vi "main.vi"() -> ()   [LabVIEW 2015]
uses:
  <vilib>/Utility/NIReport.llb/NI_report.lvclass
  Agilent 3352X Series/Agilent 3352X Series.lvlib
panel:
  out "消息":string
  in  "幅值线性度":bool=TRUE
  in  "幅频响应":bool=TRUE
  in  "参考灵敏度":bool=TRUE
  out "已连接":bool
  in  "连接设备":bool
  in  "原始记录模板":string(combo)="外接电源型加速度计(公开).xls"
  in  "被测通道":tag="PXI2Slot3/ai1:3" caption="标准通道"
  in  "方向选择":string(combo)="Z向"
  in  "参考通道":tag="PXI2Slot3/ai0" caption="标准通道"
  in  "信号发生器(33XXX系列)":refnum<visa-resource-name>="USB0::0x0957::0x2C07::MY52810975::INSTR"
  in  "保存":bool
  in  "停止":bool
  in  "测量":bool
  # "加速度传感器校准软件"
  # "仪器设置"
  # "连接"
  # "参数配置"
  # "控制"
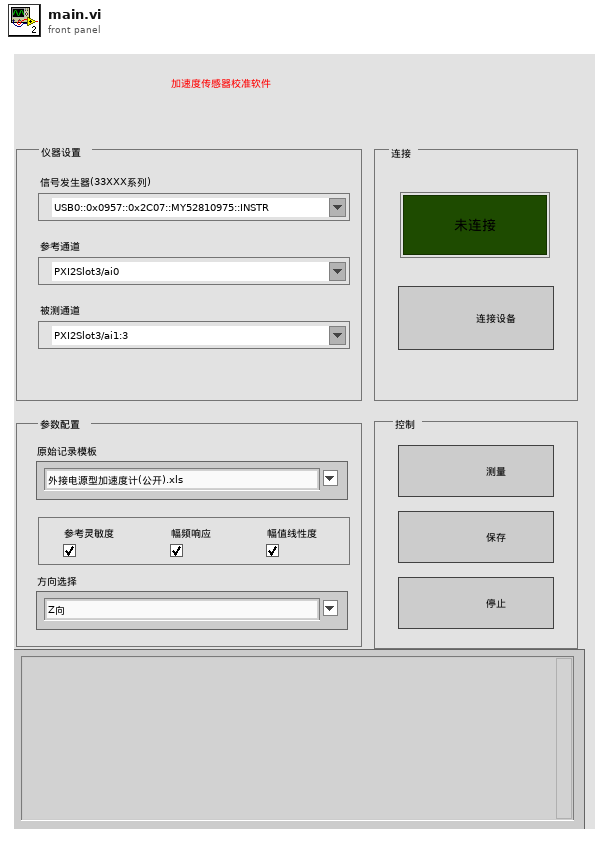
[diagram p1: front panel]
types:
  T1 = typedef "测试状态.ctl" = enum16{"idle", "路径配置", "参考灵敏度", "幅频响应", "幅值线性度", "结束", "停止"}
  T2 = typedef "句柄.ctl" = cluster{"33XXX":refnum<visa-resource-name>, "参考通道":tag, "被测通道":tag, "模板":refnum<class "NI_report.lvclass">}
  T3 = enum16{"Standard Report", "HTML", "Word", "Excel"}
  T4 = enum16{"maximized", "minimized", "normal", "no change"}
  T5 = enum8{"Enabled", "Disabled", "Disabled and Grayed Out"}
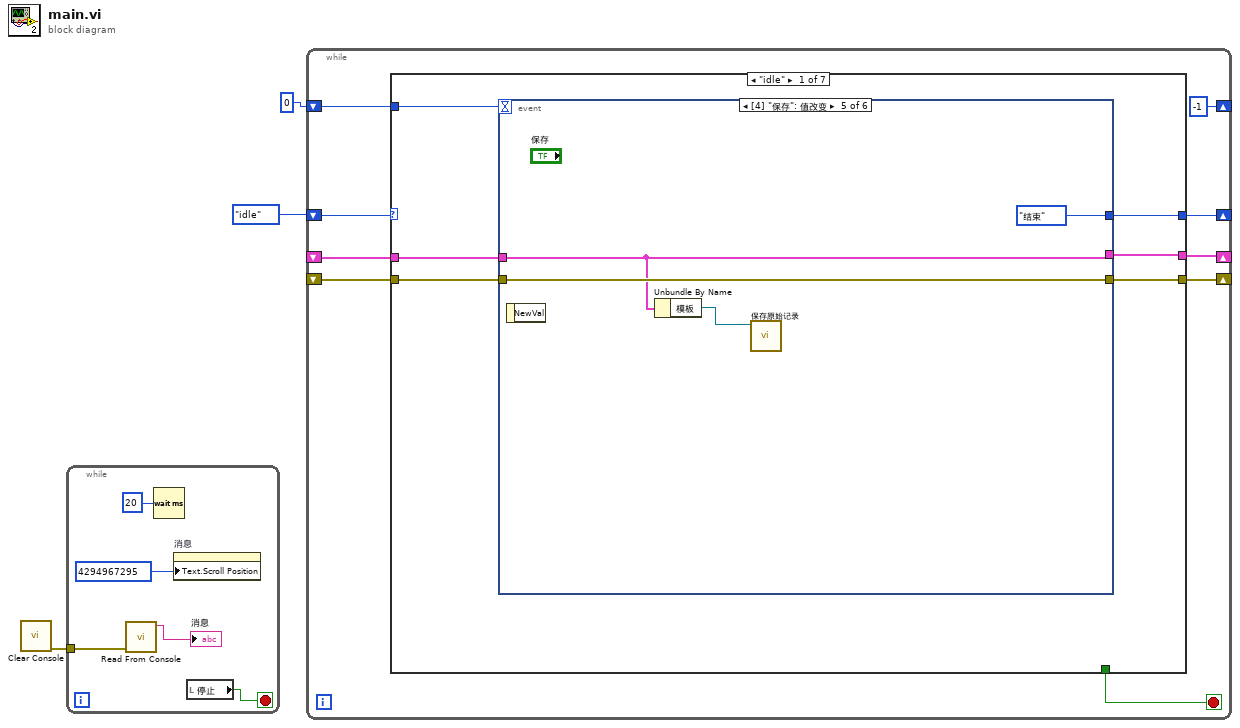
[diagram p0: block diagram]
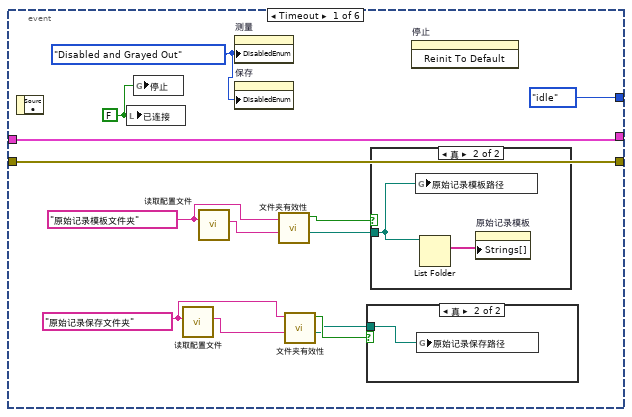
[diagram p2: hidden frame]
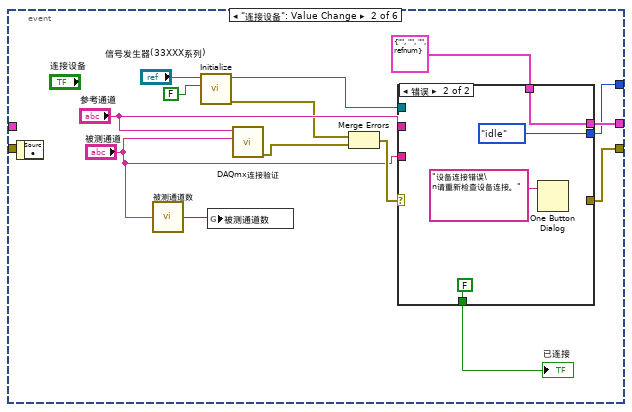
[diagram p5: hidden frame]
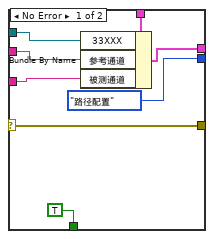
[diagram p6: hidden frame]
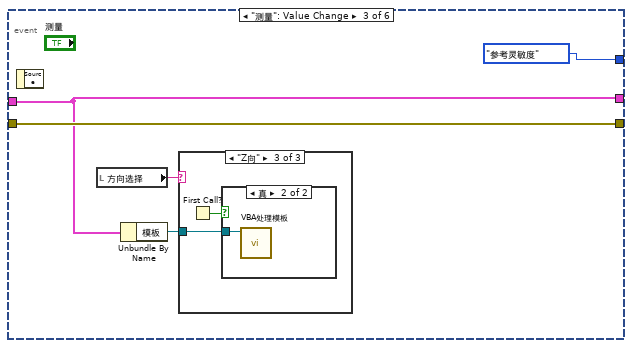
[diagram p7: hidden frame]
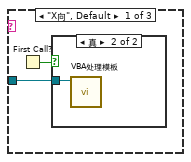
[diagram p8: hidden frame]
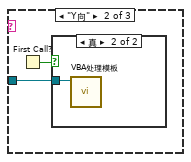
[diagram p10: hidden frame]
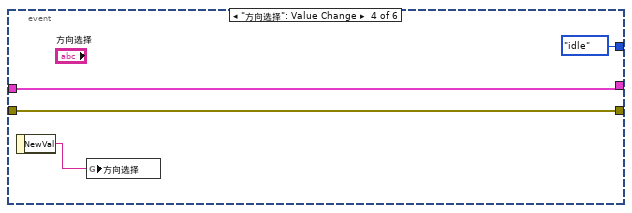
[diagram p13: hidden frame]
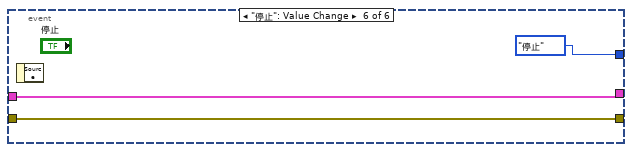
[diagram p14: hidden frame]
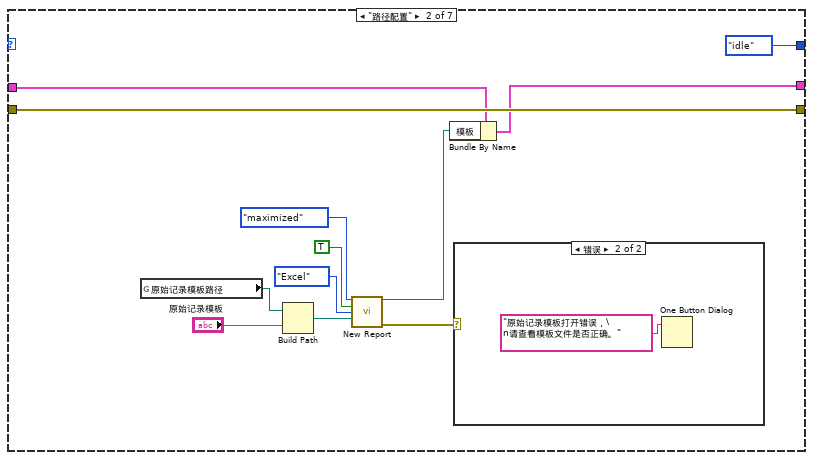
[diagram p15: hidden frame]
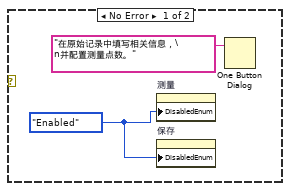
[diagram p16: hidden frame]
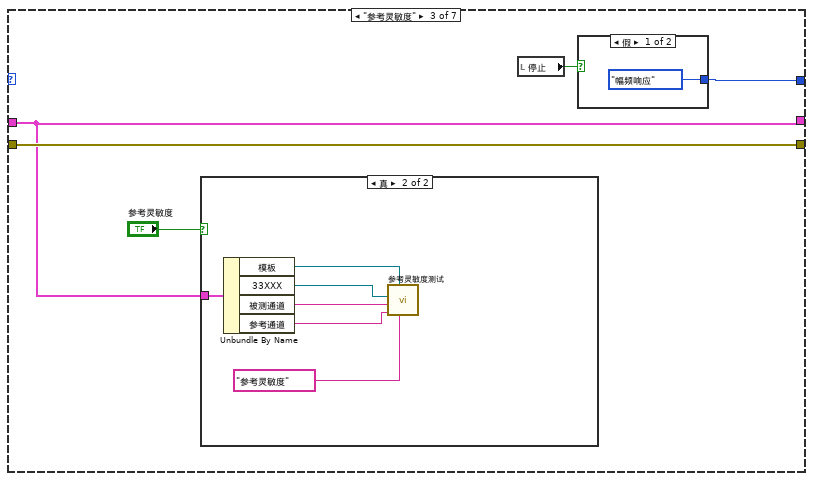
[diagram p17: hidden frame]
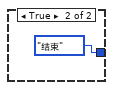
[diagram p19: hidden frame]
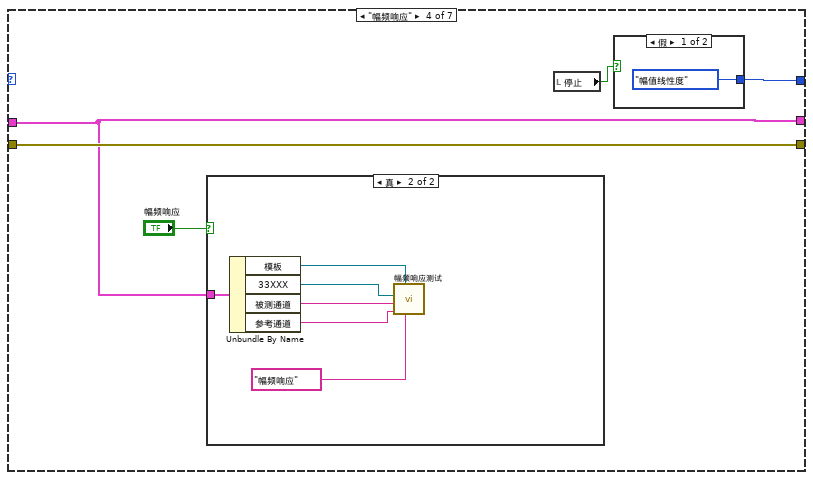
[diagram p20: hidden frame]
diagram:
  n1 = call "Clear Console.vi"() -> ("error out"=w1:errorcluster)  [unwired: 11 in]
  n2 = while {
    tunnel: w1 -> [w7]
    stop <- w4 stop-if-true
    n3 = call "Read From Console.vi"("error in (no error)"=w7) -> ("Output"=→"消息":string)  [unwired: 9 in, 1 out]
    n4 = Wait (ms)(milliseconds to wait=u32 20) -> ()  [unwired: 1 out]
    n5 = property on="消息" class="Str"("Text.Scroll Position"=u32 4294967295 ("milliseconds to wait")) -> ()  [unwired: 2 in, 2 out]
    n6 = local read "停止"() -> (w4:bool)
  }
  n7 = while {
    shift-right: [w16] -> _
    shift-left: _ -> [w14]
    shift-right: [w15] -> _
    shift-left: _ -> [w13]
    shift-right: [w12] -> _
    shift-left: 测试状态."idle" ("枚举") -> [w17]
    shift-right: [-1] -> _
    shift-left: 0 -> [w10]
    stop <- w11 stop-if-true
    n8 = case shown="\"idle\"" w17 {
      tunnel: [w23 w99 w109 w120 w133 T2 {"33XXX"="", "参考通道"="", "被测通道"="", "模板"=refnum} T2 {"33XXX"="", "参考通道"="", "被测通道"="", "模板"=refnum}] -> w16
      tunnel: [w22 w101 w110 w122 w135 w149 w158] -> w15
      tunnel: w14 -> [w21 w100 w109 w120 w133 w154 _]
      tunnel: w13 -> [w20 w101 w110 w122 w135 w152 w158]
      tunnel: [w19 测试状态."idle" ("枚举") w107 w123 测试状态."idle" ("枚举") 测试状态."idle" ("枚举") 测试状态."idle" ("枚举")] -> w12
      tunnel: [_ _ _ _ _ FALSE w157] -> w11
      tunnel: w10 -> [w18 _ _ _ _ _ _]
      frame "idle" {
        n9 = event shown="[4] \"保存\": 值改变" {
          selector: _ -> [_ _ _ _ _ _]
          dyn-events: _ -> [_ _ _ _ _ _]
          timeout: w18 -> [_ _ _ _ _ _]
          tunnel: [w36 w48 w67 w83 w85 w90] -> w23
          tunnel: [w35 w52 w70 w82 w87 w89] -> w22
          tunnel: w21 -> [w36 _ w67 w83 w85 w90]
          tunnel: w20 -> [w35 _ w70 w82 w87 w89]
          tunnel: [测试状态."idle" ("枚举") w42 测试状态."参考灵敏度" ("枚举") 测试状态."idle" ("枚举") 测试状态."结束" ("枚举") 测试状态."停止" ("枚举")] -> w19
          event Timeout {
            w25 = T5."Disabled and Grayed Out" ("禁用")
            w28 = "原始记录保存文件夹" ("配置")
            w33 = "原始记录模板文件夹" ("配置")
            w24 = FALSE ("已连接")
            n10 = event-data() -> ()  [unwired: 1 in, 1 out]
            n11 = local write "已连接"(w24) -> ()
            n12 = global write "Global.vi" "停止"(w24) -> ()
            n13 = call "读取配置文件.vi"("配置"=w28) -> ("路径"=w29:string)  [unwired: 9 in, 1 out]
            n14 = call "读取配置文件.vi"("配置"=w33) -> ("路径"=w32:string)  [unwired: 9 in, 1 out]
            n15 = property on="测量" class="Bool"("DisabledEnum"=w25) -> ()  [unwired: 2 in, 2 out]
            n16 = property on="保存" class="Bool"("DisabledEnum"=w25) -> ()  [unwired: 2 in, 2 out]
            n17 = call "文件夹有效性.vi"("路径"=w32, "配置"=w33) -> ("路径"=w31:path, "Valid"=w30:bool)  [unwired: 8 in]
            n18 = call "文件夹有效性.vi"("路径"=w29, "配置"=w28) -> ("路径"=w26:path, "Valid"=w27:bool)  [unwired: 8 in]
            n19 = case shown="真" w27 {
              tunnel: w26 -> [_ w37]
              frame False {
              }
              frame True {
                n20 = global write "Global.vi" "原始记录保存路径"(w37) -> ()
              }
            }
            n21 = case shown="真" w30 {
              tunnel: w31 -> [_ w39]
              frame False {
              }
              frame True {
                n22 = global write "Global.vi" "原始记录模板路径"(w39) -> ()
                n23 = List Folder(path=w39) -> (filenames=w38:string[])  [unwired: 3 in, 3 out]
                n24 = property on="原始记录模板" class="CmbBox"("Strings[]"=w38) -> ()  [unwired: 2 in, 2 out]
              }
            }
            n25 = invoke on="停止" class="Bool (严格)" method="Reinit To Default"() -> ()  [unwired: 3 in, 3 out]
          }
          event "连接设备": Value Change {
            n26 = event-data() -> ()  [unwired: 1 in, 1 out]
            n27 = call "被测通道数.vi"("被测通道"="被测通道") -> ("被测通道数"=w40:i32)
            n28 = call "Initialize.vi"("ID Query (Enable)"=FALSE ("ID Query (True)"), "VISA resource name"="信号发生器(33XXX系列)") -> ("error out"=w43:errorcluster, "VISA resource name out"=w44:refnum<visa-resource-name>)  [unwired: 8 in]
            n29 = global write "Global.vi" "被测通道数"(w40) -> ()
            n30 = call "DAQmx连接验证.vi"("被测"="被测通道", "参考"="参考通道") -> ("error out"=w50:errorcluster)  [unwired: 9 in]
            n31 = Merge Errors(w43, w50) -> (w53:errorcluster)
            n32 = case shown="错误" w53 {
              selector: w53 -> [w60 _]
              tunnel: w44 -> [w61 _]
              tunnel: "参考通道" -> [w58 _]
              tunnel: [w57 w63] -> w48
              tunnel: [w60 _] -> w52
              tunnel: [TRUE FALSE ("已连接")] -> w51
              tunnel: "被测通道" -> [w56 _]
              tunnel: T2 {"33XXX"="", "参考通道"="", "被测通道"="", "模板"=refnum} -> [w55 w63]
              tunnel: [测试状态."路径配置" ("枚举") 测试状态."idle" ("枚举")] -> w42
              frame No Error {
                n33 = Bundle By Name(cluster=w55, "33XXX"=w61, "参考通道"=w58, "被测通道"=w56) -> (w57:T2)
              }
              frame Error {
                n34 = One Button Dialog(message="设备连接错误\n请重新检查设备连接。") -> ()  [unwired: 1 in, 1 out]
              }
            }
            "已连接" <- w51
          }
          event "测量": Value Change {
            n35 = event-data() -> ()  [unwired: 1 in, 1 out]
            n36 = local read "方向选择"() -> (w68:string)
            n37 = Unbundle By Name(w67) -> ("模板"=w66:refnum<class "NI_report.lvclass">)
            n38 = case shown="\"Z向\"" w68 {
              tunnel: w66 -> [w71 w74 w77]
              frame "X向", Default {
                n39 = First Call?() -> (First Call?: T/F=w72:bool)
                n40 = case shown="真" w72 {
                  tunnel: w71 -> [_ w73]
                  frame False {
                  }
                  frame True {
                    n41 = call "VBA处理模板.vi"("NI_report输入"=w73) -> ()  [unwired: 10 in, 1 out]
                  }
                }
              }
              frame "Y向" {
                n42 = First Call?() -> (First Call?: T/F=w75:bool)
                n43 = case shown="真" w75 {
                  tunnel: w74 -> [_ w76]
                  frame False {
                  }
                  frame True {
                    n44 = call "VBA处理模板.vi"("NI_report输入"=w76) -> ()  [unwired: 10 in, 1 out]
                  }
                }
              }
              frame "Z向" {
                n45 = First Call?() -> (First Call?: T/F=w78:bool)
                n46 = case shown="真" w78 {
                  tunnel: w77 -> [_ w79]
                  frame False {
                  }
                  frame True {
                    n47 = call "VBA处理模板.vi"("NI_report输入"=w79) -> ()  [unwired: 10 in, 1 out]
                  }
                }
              }
            }
          }
          event "方向选择": Value Change {
            n48 = event-data() -> ("NewVal"=w80:string)  [unwired: 1 in]
            n49 = global write "Global.vi" "方向选择"(w80) -> ()
          }
          event "保存": Value Change {
            n50 = event-data() -> ()  [unwired: 1 in, 1 out]
            n51 = Unbundle By Name(w85) -> ("模板"=w84:refnum<class "NI_report.lvclass">)
            n52 = call "保存原始记录.vi"("NI_report输入"=w84) -> ()  [unwired: 10 in, 1 out]
          }
          event "停止": Value Change {
            n53 = event-data() -> ()  [unwired: 1 in, 1 out]
          }
        }
      }
      frame "路径配置" {
        n54 = global read "Global.vi" "原始记录模板路径"() -> (w94:path)
        n55 = Build Path(base path=w94, name or relative path="原始记录模板") -> (appended path=w98:path)
        n56 = call <vilib>:"New Report.vi"("window state (normal)"=T4."maximized", "display alerts? (F)"=TRUE, "report type"=T3."Excel", "template (empty)"=w98) -> ("report out"=w92:refnum<class "NI_report.lvclass">, "error out"=w91:errorcluster)  [unwired: 10 in]
        n57 = Bundle By Name(cluster=w100, "模板"=w92) -> (w99:T2)
        n58 = case shown="错误" w91 {
          frame No Error {
            w103 = T5."Enabled" ("禁用")
            n59 = property on="测量" class="Bool"("DisabledEnum"=w103) -> ()  [unwired: 2 in, 2 out]
            n60 = property on="保存" class="Bool"("DisabledEnum"=w103) -> ()  [unwired: 2 in, 2 out]
            n61 = One Button Dialog(message="在原始记录中填写相关信息，\n并配置测量点数。" ("消息")) -> ()  [unwired: 1 in, 1 out]
          }
          frame Error {
            n62 = One Button Dialog(message="原始记录模板打开错误，\n请查看模板文件是否正确。" ("消息")) -> ()  [unwired: 1 in, 1 out]
          }
        }
      }
      frame "参考灵敏度" {
        n63 = case shown="真" "参考灵敏度" {
          tunnel: w109 -> [_ w116]
          frame False {
          }
          frame True {
            n64 = Unbundle By Name(w116) -> ("模板"=w115:refnum<class "NI_report.lvclass">, "33XXX"=w114:refnum<visa-resource-name>, "被测通道"=w113:tag, "参考通道"=w112:tag)
            n65 = call "参考灵敏度测试.vi"("参数"="参考灵敏度", "模板"=w115, "参考通道"=w112, "被测通道"=w113, "33XXX"=w114) -> ()  [unwired: 6 in, 1 out]
          }
        }
        n66 = local read "停止"() -> (w108:bool)
        n67 = case shown="假" w108 {
          tunnel: [测试状态."幅频响应" ("枚举") 测试状态."结束" ("枚举")] -> w107
          frame False {
          }
          frame True {
          }
        }
      }
      frame "幅频响应" {
        n68 = case shown="真" "幅频响应" {
          tunnel: w120 -> [_ w129]
          frame False {
          }
          frame True {
            n69 = Unbundle By Name(w129) -> ("模板"=w128:refnum<class "NI_report.lvclass">, "33XXX"=w127:refnum<visa-resource-name>, "被测通道"=w126:tag, "参考通道"=w125:tag)
            n70 = call "幅频响应测试.vi"("参数"="幅频响应", "模板"=w128, "参考通道"=w125, "被测通道"=w126, "33XXX"=w127) -> ()  [unwired: 6 in, 1 out]
          }
        }
        n71 = local read "停止"() -> (w121:bool)
        n72 = case shown="假" w121 {
          tunnel: [测试状态."幅值线性度" ("枚举") 测试状态."结束" ("枚举")] -> w123
          frame False {
          }
          frame True {
          }
        }
      }
      frame "幅值线性度" {
        n73 = case shown="真" "幅值线性度" {
          tunnel: w133 -> [_ w138]
          tunnel: [_ w137] -> w132
          frame False {
          }
          frame True {
            n74 = Unbundle By Name(w138) -> ("模板"=w143:refnum<class "NI_report.lvclass">, "33XXX"=w142:refnum<visa-resource-name>, "被测通道"=w141:tag, "参考通道"=w140:tag)
            n75 = call "幅值线性度测试.vi"("参数"="幅值线性度", "模板"=w143, "参考通道"=w140, "被测通道"=w141, "33XXX"=w142) -> ("错误输出"=w137:errorcluster)  [unwired: 6 in]
          }
        }
        n76 = flat-sequence {
          tunnel: w132 -> [_]
          frame #0 {
            n77 = global read "Global.vi" "方向选择"() -> (w148:string)
            n78 = Concatenate Strings("“" ("字符串"), w148, "”测量完成。" ("字符串"), "\r\n") -> (w145:string)
            n79 = One Button Dialog(message=w145) -> ()  [unwired: 1 in, 1 out]
            n80 = call "Write to Console.vi"("Input"=w145) -> ()  [unwired: 10 in, 1 out]
          }
        }
      }
      frame "结束" {
        n81 = Unbundle By Name(w154) -> ("33XXX"=w153:refnum<visa-resource-name>)
        n82 = local write "已连接"(FALSE ("已连接")) -> ()
        n83 = call "Close.vi"("error in (no error)"=w152, "VISA resource name"=w153) -> ("error out"=w149:errorcluster)  [unwired: 9 in]
      }
      frame "停止" {
        w157 = TRUE
        n84 = global write "Global.vi" "停止"(w157) -> ()
      }
    }
  }
